vi "terminate.vi"(8 "error in (no error)":errorcluster, 11 "GenericPlugin in":refnum<class "StageMH110930Scientifica.lvclass">) -> (0 "error out":errorcluster, 3 "GenericPlugin out":refnum<class "StageMH110930Scientifica.lvclass">)   [LabVIEW 2010, in "StageMH110930Scientifica.lvclass"]
doc: "The dynamic dispatch version of this VI terminates the plug-in object by releasing all of its resources."
uses:
  StageMH110930Scientifica.lvclass
  StageDL090409Scaffold/StageDL090409Scaffold/StageDL090409Scaffold.lvclass
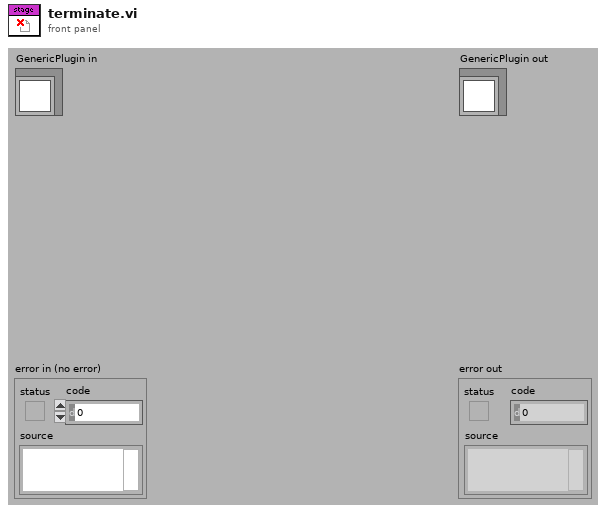
[diagram p1: front panel]
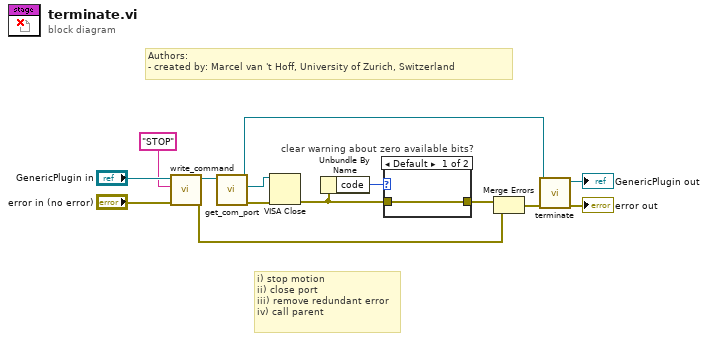
[diagram p0: block diagram]
diagram:
  # "i) stop motion\nii) close port\niii) remove redundant error\niv) call parent"
  # "Authors: \n- created by: Marcel van 't Hoff, University of Zurich, Switzerland"
  n1 = call-dynamic "write_command.vi"("error in (no error)"="error in (no error)", "string to write"="STOP", "StageMH110930Scientifica in"="GenericPlugin in") -> ("error out"=w2:errorcluster, "StageMH110930Scientifica out"=w1:refnum<class "StageMH110930Scientifica.lvclass">)  [unwired: 5 in, 2 out]
  n2 = call-dynamic "get_com_port.vi"("StageMH110930Scientifica in"=w1) -> ("error out"=w11:errorcluster, "serial port name"=w12:refnum<visa-resource-name>, "StageMH110930Scientifica out"=w10:refnum<class "StageMH110930Scientifica.lvclass">)  [unwired: 8 in]
  n3 = VISA Close(VISA resource name=w12, error in (no error)=w11) -> (error out=w7:errorcluster)
  n4 = Unbundle By Name(w7) -> ("code"=w8:i32)
  n5 = case "clear warning about zero available bits?" shown="Default" w8 {
    tunnel: [w15 _] -> w6
    tunnel: w7 -> [w15 _]
    frame Default {
    }
    frame 1073676294 {
    }
  }
  n6 = Merge Errors(w6, w2) -> (w9:errorcluster)
  n7 = call-parent "terminate.vi"("error in (no error)"=w9, "GenericPlugin in"=w10) -> ("error out"=→"error out":errorcluster, "GenericPlugin out"=→"GenericPlugin out":refnum<class "StageMH110930Scientifica.lvclass">)  [unwired: 8 in]
